vi "main.vi"() -> ()   [LabVIEW 2020]
panel:
  out "Wash Entry":bool
  in  "Stop":bool
  in  "Wash Options":T1
  in  "Start":bool
  out "Elapsed Time":dbl format="%.2f"
  out "Car Wash Indicators":T2
  in  "Car Position Slider":u8(slide) scale=0.0..4.0
  # "Entry Console"
  # "Car Wash Display"
  # "Car Position Simulation"
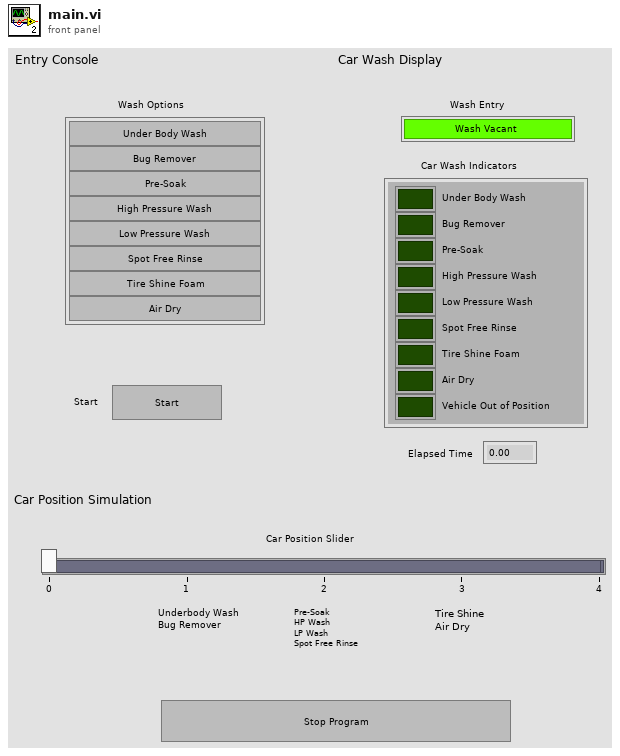
[diagram p1: front panel]
types:
  T1 = cluster{"Under Body Wash":bool, "Bug remover":bool, "Pre-soak":bool, "High Pressure Wash":bool, "Low Pressure Wash":bool, "Spot Free Rinse":bool, "Tire Shine Foam":bool, "Air Dry":bool}
  T2 = cluster{"Under Body Wash":bool, "Bug Remover":bool, "Pre-Soak":bool, "High Pressure Wash":bool, "Low Pressure Wash":bool, "Spot Free Rinse":bool, "Tire Shine Foam":bool, "Air Dry":bool, "Vehicle Out of Position":bool}
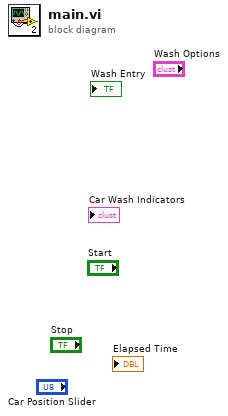
[diagram p0: block diagram]
diagram:
